vi "TCP-Read Data Out.vi"(8 "error in":errorcluster, 10 "TCP-IP Data Out":string, 11 "Module ID":i32=-1) -> (0 "error out":errorcluster)   [LabVIEW 2018, in "TCP-IP Engine.lvlib"]
doc: "This Broadcast Event will send the Data which has been read from the TCP-IP Conection.\n_____\nCreated using DQMH Event Scripter 7.0.1.1316."
uses:
  TCP-IP Engine.lvlib
  TCP-Read Data Out Argument--cluster.ctl
  <vilib>/event_ctls.llb/usereventprio.ctl
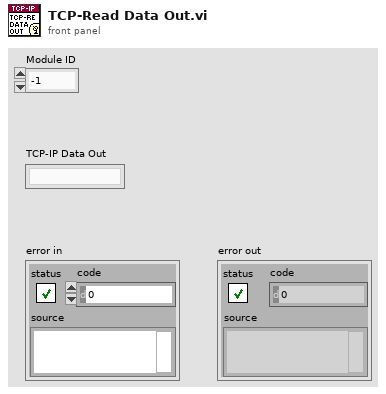
[diagram p1: front panel]
types:
  T1 = typedef "usereventprio.ctl" = enum32{"high priority", "normal priority"}
  T2 = typedef "TCP-IP Engine.lvlib/TCP-Read Data Out Argument--cluster.ctl" = cluster{"Module ID":i32, "TCP-IP Data Out":string}
  T3 = typedef "TCP-IP Engine.lvlib/Broadcast Events--cluster.ctl" = cluster{"Module Did Init":refnum<user-event>, "Status Updated":refnum<user-event>, "Error Reported":refnum<user-event>, "Module Did Stop":refnum<user-event>, "Update Module Execution Status":refnum<user-event>, "Open Connection Status":refnum<user-event>, "TCP-Read Data Out":refnum<user-event>}
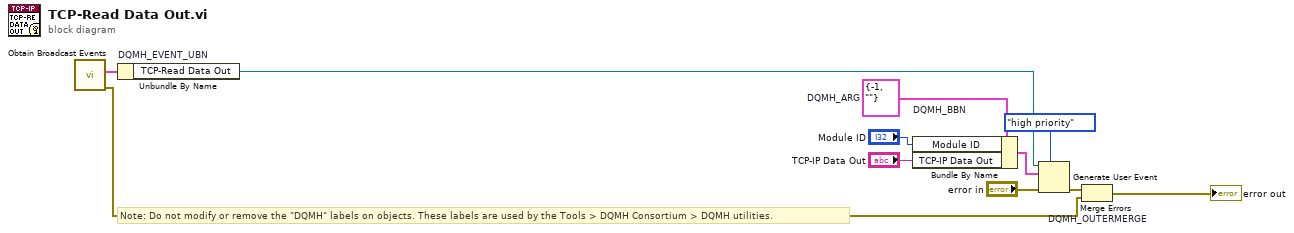
[diagram p0: block diagram]
diagram:
  w6 = T2 {"Module ID"=-1, "TCP-IP Data Out"=""}  # DQMH_ARG
  # "Note: Do not modify or remove the \"DQMH\" labels on objects. These labels are used by the Tools > DQMH Consortium > DQMH utilities."
  n1 = call "Obtain Broadcast Events.vi"() -> ("error out"=w3:errorcluster, "TCP-IP Engine Broadcast Events"=w2:T3)  [unwired: 10 in]
  n2 = Unbundle By Name "DQMH_EVENT_UBN"(w2) -> ("TCP-Read Data Out"=w8:refnum<user-event>)
  n3 = Bundle By Name "DQMH_BBN"(cluster=w6, "Module ID"="Module ID", "TCP-IP Data Out"="TCP-IP Data Out") -> (w9:T2)
  n4 = Generate User Event(priority (normal)=usereventprio."high priority", user event=w8, event data cluster=w9, error in="error in") -> (error out=w7:errorcluster)  [unwired: 1 out]
  n5 = Merge Errors "DQMH_OUTERMERGE"(w7, w3) -> (→"error out":errorcluster)
